vi "PH_Beckhoff_PPMA-Rods.get Rods Tagname.vi"(1 "Rods Tag":T1) -> (0 "Rods Tagname":string)   [LabVIEW 2014, in "PH_Beckhoff_PPMA-Rods.lvlib"]
doc: "This VI concatenates a Tagname out of strict type def enum controls. It keeps also the information whether the Tag is existing (if not, N/A is given out as name)."
uses:
  PH_Beckhoff_PPMA-Rods.lvlib
  PH_Beckhoff_PPMA-Rods.Rods Tags.ctl
  PH_Basics/PH_Common/Names/PH_Names.Subsystems.ctl
  PH_Basics/PH_PP_Common/PH_PP_Common.Devices.ctl
  PH_Basics/PH_Common/Names/PH_Names.Communication Type.ctl
  PH_Basics/PH_Common/PH_Common.lvlib
  PH_Basics/PH_PP_Common/PH_PP_Common.lvlib
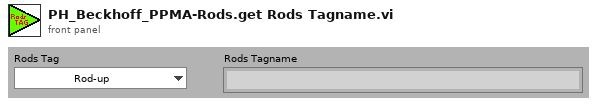
[diagram p1: front panel]
types:
  T1 = typedef "PH_Beckhoff_PPMA-Rods.lvlib/PH_Beckhoff_PPMA-Rods.Rods Tags.ctl" = enum16{"Rod-up", "earth-ok", "door-locked-K1", "door-locked-K2", "watervalve-closed", "Rods-Chain-A-up", "Rods-Chain-B-up", "HV-Warnlamp-orange", "HV-Warnlamp-green", "Status-Rods-PU-1", "Status-Rods-PU-2", "Status-Rods-PU-3", "Status-Rods-PU-4", "Status-Rods-PU-5", "Status-Rods-PU-6", "Status-Rods-PU-7", "Status-Rods-PU-8", "Status-Rods-PU-9", "Status-Rods-PU-10", "Status-Rods-FR", "Status-Rods-PILC"}
  T2 = typedef "PH_PP_Common.lvlib/PH_PP_Common.Devices.ctl" = enum16{"no Info", "Igni", "RR", "DumpRoss", "PSU", "Trigger", "HV-Meas", "Rods", "Chiller", "Conductivity", "Mercury"}
  T3 = typedef "PH_Common.lvlib/PH_Names.Subsystems.ctl" = enum16{"no Info", "fs-FE", "ns-FE", "PA", "MA", "MAS", "COS", "Exp-LB", "Exp-LL", "PP", "PILS"}
  T4 = typedef "PH_Common.lvlib/PH_Names.Communication Type.ctl" = enum16{"no Info", "SE", "SA", "AE", "AA", "DE", "DA", "DIM"}
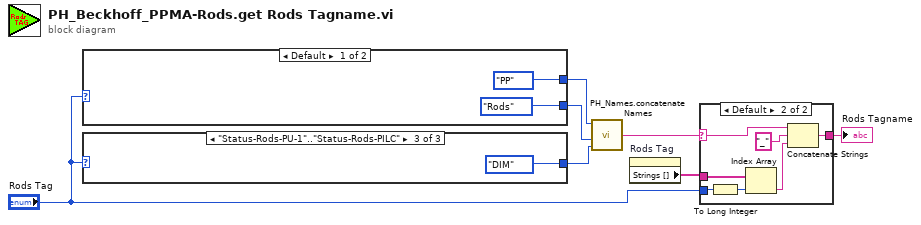
[diagram p0: block diagram]
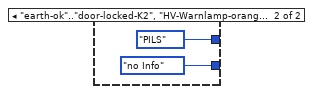
[diagram p2: hidden frame]
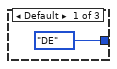
[diagram p3: hidden frame]
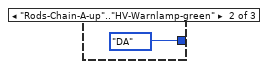
[diagram p4: hidden frame]
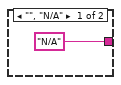
[diagram p5: hidden frame]
diagram:
  n1 = case shown="Default" "Rods Tag" {
    tunnel: [PH_Names.Subsystems."PP" ("Subsystem") PH_Names.Subsystems."PILS" ("Subsystem")] -> w3
    tunnel: [PH_PP_Common.Devices."Rods" ("Devices (no info)") PH_PP_Common.Devices."no Info" ("Devices (no info)")] -> w2
    frame Default {
    }
    frame "earth-ok".."door-locked-K2", "HV-Warnlamp-orange", "HV-Warnlamp-green" {
    }
  }
  n2 = case shown="\"Status-Rods-PU-1\"..\"Status-Rods-PILC\"" "Rods Tag" {
    tunnel: [PH_Names.Communication_Type."DE" ("Communication Type (no info)") PH_Names.Communication_Type."DA" ("Communication Type (no info)") PH_Names.Communication_Type."DIM" ("Communication Type (no info)")] -> w4
    frame Default {
    }
    frame "Rods-Chain-A-up".."HV-Warnlamp-green" {
    }
    frame "Status-Rods-PU-1".."Status-Rods-PILC" {
    }
  }
  n3 = call "PH_Names.concatenate Names.vi"("Communication Type (no info)"=w4, "Devices (no info)"=w2, "Subsystem"=w3) -> ("Subsystem_PU_Devices_Comm Type"=w6:string)  [unwired: 1 in]
  n4 = property on="Rods Tag" class="Enum (strict)"() -> ("Strings []"=w5:string[])  [unwired: 2 in, 2 out]
  n5 = case shown="Default" w6 {
    selector: w6 -> [_ w16]
    tunnel: ["N/A" w22] -> w7
    tunnel: w5 -> [_ w21]
    tunnel: "Rods Tag" -> [_ w17]
    frame "", "N/A" {
    }
    frame Default {
      n6 = To Long Integer(number=w17) -> (32bit integer=w20:i32)
      n7 = Index Array(array=w21, index=w20) -> (element=w19:string)
      n8 = Concatenate Strings(w16, "_" ("string"), w19) -> (w22:string)
    }
  }
  "Rods Tagname" <- w7
